vi "OBJ_evaluate_result.vi"(9 "high_limit":string, 10 "measurement":string, 11 "low_limit":string) -> (1 "OK?":bool, 2 "status":T1, 3 "status_string":string)   [LabVIEW 2019]
uses:
  OBJ_measurement_status.ctl
  _misc/AULocalize/SubVIs/Get Localized Phrase Compact Interface 0D.vi
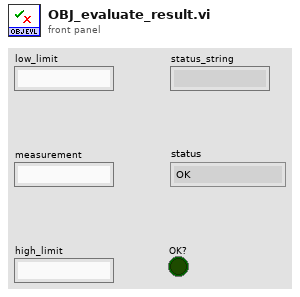
[diagram p1: front panel]
types:
  T1 = typedef "OBJ_measurement_status.ctl" = enum16{"OK", "NOK"}
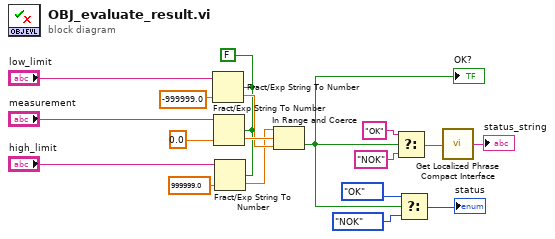
[diagram p0: block diagram]
diagram:
  w5 = FALSE ("use system decimal point (T)")
  n1 = Fract/Exp String To Number(use system decimal point (T)=w5, string="low_limit", default (0 dbl)=sgl -999999.0 ("default (0 DBL)")) -> (number=w7:sgl)  [unwired: 1 in, 1 out]
  n2 = Fract/Exp String To Number(use system decimal point (T)=w5, string="measurement", default (0 dbl)=sgl 0.0 ("default (0 DBL)")) -> (number=w8:sgl)  [unwired: 1 in, 1 out]
  n3 = Fract/Exp String To Number(use system decimal point (T)=w5, string="high_limit", default (0 dbl)=sgl 999999.0 ("default (0 DBL)")) -> (number=w6:sgl)  [unwired: 1 in, 1 out]
  n4 = In Range and Coerce(upper limit=w6, x=w8, lower limit=w7) -> (In Range?=w17:bool)  [unwired: 1 out]
  "OK?" <- w17
  n5 = Select(t="OK", s=w17, f="NOK") -> (s? t:f=w14:string)
  n6 = Select(t=OBJ_measurement_status."OK" ("SQL_connection_status"), s=w17, f=OBJ_measurement_status."NOK" ("SQL_connection_status")) -> (s? t:f=→"status":T1)
  n7 = call-poly "Get Localized Phrase Compact Interface.vi"("Key"=w14) -> ("Translated Phrase"=→"status_string":string)
